vi "Get-client-channel-by-id.vi"(8 "error in (no error)":errorcluster, 10 "Client ID":i32, 11 "ModComm in":T1) -> (0 "error out":errorcluster, 2 "Client channel":refnum<queue>, 3 "ModComm out":T1)   [LabVIEW 2013, in "Server.lvlib" / "Server.lvclass"]
uses:
  Server.lvclass
  Object-reference.ctl
  Messages/Sources/Message.lvclass
  Server.lvclass/Server.ctl
  Read Client channels.vi
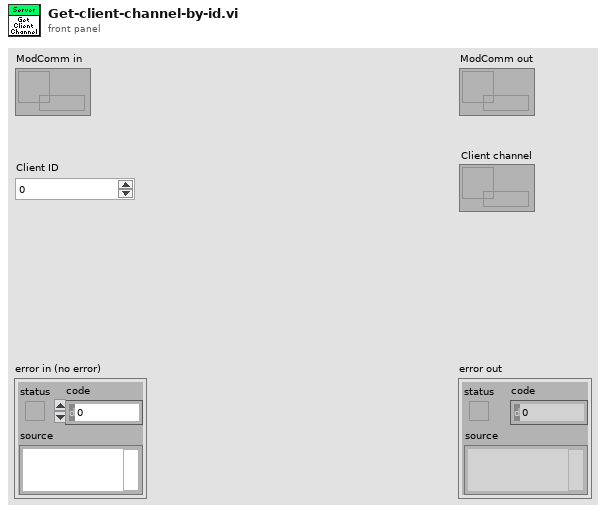
[diagram p1: front panel]
types:
  T1 = typedef "Server.lvlib/Server.lvclass/Object-reference.ctl" = refnum<data-value>
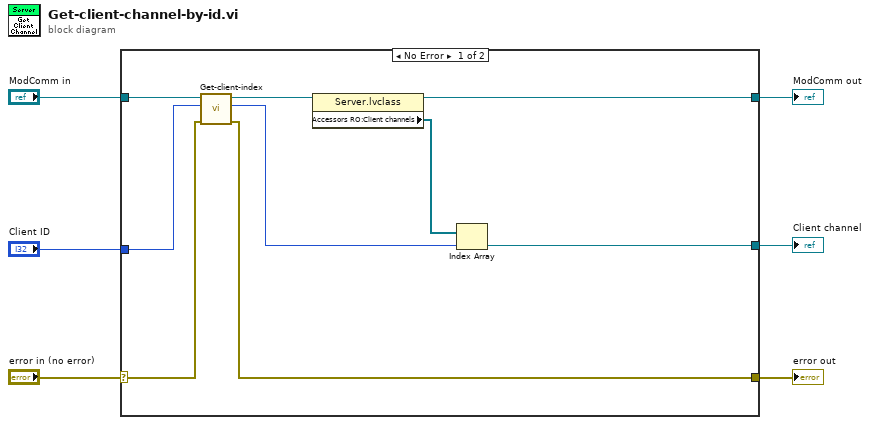
[diagram p0: block diagram]
diagram:
  n1 = case shown="No Error" "error in (no error)" {
    selector: "error in (no error)" -> [w12 w17]
    tunnel: [w11 w17] -> w5
    tunnel: [w15 w16] -> w3
    tunnel: "ModComm in" -> [w14 w16]
    tunnel: "Client ID" -> [w10 _]
    tunnel: [w7 _] -> w1
    frame No Error {
      n2 = call "Get-client-index.vi"("error in (no error)"=w12, "Client ID"=w10, "ModComm in"=w14) -> ("error out"=w11:errorcluster, "Client index"=w8:i32, "ModComm out"=w13:T1)  [unwired: 6 in]
      n3 = property class="Server.lvclass"(reference=w13) -> (reference out=w15:T1, "Accessors RO:Client channels"=w9:refnum<queue>[])  [unwired: 1 in, 1 out]
      n4 = Index Array(array=w9, index=w8) -> (element=w7:refnum<queue>)
    }
    frame Error {
    }
  }
  "error out" <- w5
  "ModComm out" <- w3
  "Client channel" <- w1
